vi "Start Reader.vi"(8 "error in (no error)":errorcluster, 11 "CAN_Logic in":refnum<class "CAN_Logic.lvclass">) -> (0 "error out":errorcluster, 3 "CAN_Logic out":refnum<class "CAN_Logic.lvclass">)   [LabVIEW 2021, in "CAN_Logic.lvclass"]
uses:
  CAN_Logic.lvclass
  CAN_Logic.lvclass/CAN_Logic.ctl
  <vilib>/xnet/xnet.llb/XNET Create Session (Frame Input Stream).vi
  <resource>/objmgr/xnet.rc
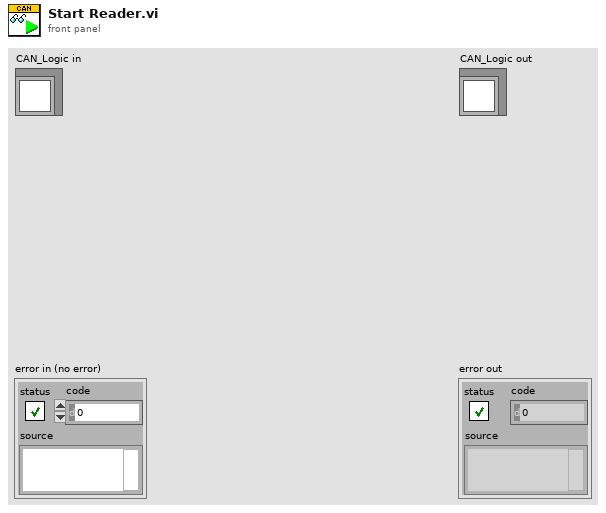
[diagram p1: front panel]
types:
  T1 = typedef "CAN_Logic.lvclass/FD Config.ctl" = cluster{"FD Baud Rate":u64, "ISO Mode":bool, "BRS Enabled":bool}
  T2 = typedef "CAN_Logic.lvclass/CAN Mode.ctl" = enum16{"CAN 2.0", "CAN FD"}
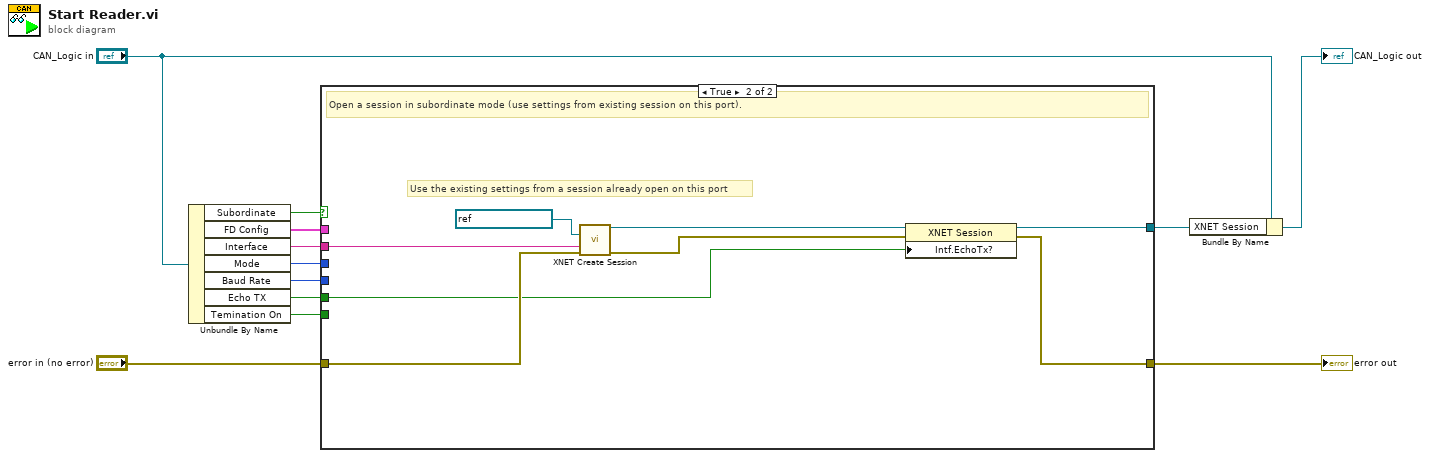
[diagram p0: block diagram]
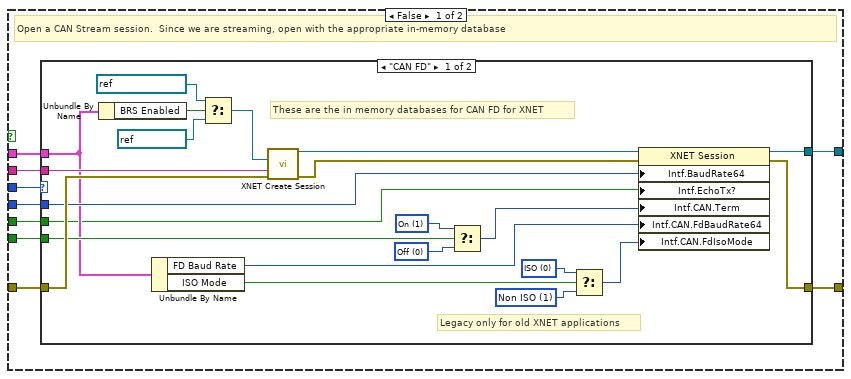
[diagram p2: hidden frame]
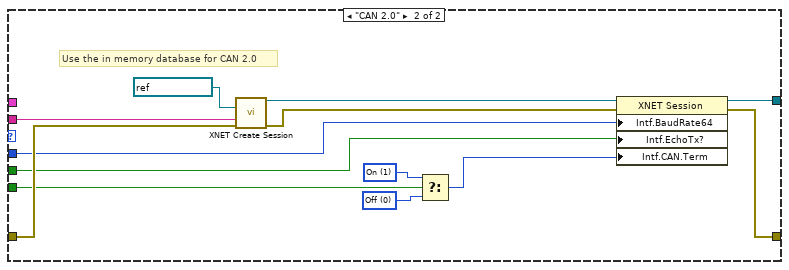
[diagram p3: hidden frame]
diagram:
  n1 = Unbundle By Name("CAN_Logic in") -> ("Subordinate"=w5:bool, "FD Config"=w9:T1, "Interface"=w12:string, "Mode"=w8:T2, "Baud Rate"=w10:u64, "Echo TX"=w1:bool, "Temination On"=w2:bool)
  n2 = case shown="True" w5 {
    tunnel: w12 -> [w21 w64]
    tunnel: "error in (no error)" -> [w20 w63]
    tunnel: w10 -> [w19 _]
    tunnel: w2 -> [w18 _]
    tunnel: w9 -> [w17 _]
    tunnel: w8 -> [w16 _]
    tunnel: [w15 w60] -> w4
    tunnel: [w14 w58] -> w3
    tunnel: w1 -> [w13 w57]
    frame False {
      # "Open a CAN Stream session.  Since we are streaming, open with the appropriate in-memory database"
      n3 = case shown="\"CAN FD\"" w16 {
        tunnel: w21 -> [w43 w56]
        tunnel: w20 -> [w42 w55]
        tunnel: w19 -> [w34 w50]
        tunnel: w18 -> [w35 w51]
        tunnel: w17 -> [w31 _]
        tunnel: [w26 w48] -> w14
        tunnel: [w25 w47] -> w15
        tunnel: w13 -> [w22 w45]
        frame "CAN FD" {
          w28 = u32 1 items=["ISO", "Non ISO", "ISO Legacy"] ("Interface:CAN:FD ISO Mode")
          w29 = u32 0 items=["ISO", "Non ISO", "ISO Legacy"] ("Interface:CAN:FD ISO Mode")
          w33 = u32 0 items=["Off", "On"] ("Interface:CAN:Termination")
          w37 = u32 1 items=["Off", "On"] ("Interface:CAN:Termination")
          # "These are the in memory databases for CAN FD for XNET"
          # "Legacy only for old XNET applications"
          n4 = Unbundle By Name(w31) -> ("BRS Enabled"=w32:bool)
          n5 = Unbundle By Name(w31) -> ("FD Baud Rate"=w24:u64, "ISO Mode"=w30:bool)
          n6 = Select(t=refnum<k21> ":can_fd_brs:" ("cluster (:memory:)"), s=w32, f=refnum<k21> ":can_fd:" ("cluster (:memory:)")) -> (s? t:f=w39:refnum<k21>)
          n7 = call-poly <vilib>:"XNET Create Session.vi"("cluster (:memory:)"=w39, "interface"=w43, "error in (no error)"=w42) -> ("session out"=w38:refnum<k21>, "error out"=w36:errorcluster)  [unwired: 11 in]
          n8 = Select(t=w37, s=w35, f=w33) -> (s? t:f=w23:u32)
          n9 = Select(t=w29, s=w30, f=w28) -> (s? t:f=w27:u32)
          n10 = property class="XNET Session"(reference=w38, error in=w36, "Intf.BaudRate64"=w34, "Intf.EchoTx?"=w22, "Intf.CAN.Term"=w23, "Intf.CAN.FdBaudRate64"=w24, "Intf.CAN.FdIsoMode"=w27) -> (reference out=w25:refnum<k21>, error out=w26:errorcluster)
        }
        frame "CAN 2.0" {
          w49 = u32 0 items=["Off", "On"] ("Interface:CAN:Termination")
          w53 = u32 1 items=["Off", "On"] ("Interface:CAN:Termination")
          # "Use the in memory database for CAN 2.0"
          n11 = call-poly <vilib>:"XNET Create Session.vi"("cluster (:memory:)"=refnum<k21> ":memory:", "interface"=w56, "error in (no error)"=w55) -> ("session out"=w54:refnum<k21>, "error out"=w52:errorcluster)  [unwired: 11 in]
          n12 = Select(t=w53, s=w51, f=w49) -> (s? t:f=w46:u32)
          n13 = property class="XNET Session"(reference=w54, error in=w52, "Intf.BaudRate64"=w50, "Intf.EchoTx?"=w45, "Intf.CAN.Term"=w46) -> (reference out=w47:refnum<k21>, error out=w48:errorcluster)
        }
      }
    }
    frame True {
      # "Use the existing settings from a session already open on this port"
      # "Open a session in subordinate mode (use settings from existing session on this port)."
      n14 = call-poly <vilib>:"XNET Create Session.vi"("cluster (:memory:)"=refnum<k21> ":subordinate:", "interface"=w64, "error in (no error)"=w63) -> ("session out"=w61:refnum<k21>, "error out"=w59:errorcluster)  [unwired: 11 in]
      n15 = property class="XNET Session"(reference=w61, error in=w59, "Intf.EchoTx?"=w57) -> (reference out=w60:refnum<k21>, error out=w58:errorcluster)
    }
  }
  "error out" <- w3
  n16 = Bundle By Name(cluster="CAN_Logic in", "XNET Session"=w4) -> (→"CAN_Logic out":refnum<class "CAN_Logic.lvclass">)
